vi "sn_To_Project.vi"(11 "s/n":string) -> (3 "project":string)   [LabVIEW 2011]
panel:
  in  "SerialNumber":string="[)> 06 1PLA18CB0-B40K000-F W480666 S54065 10D2047"
  # "To908.vi\nPassword:Abcd1234*\n20221117:Start new version for build Short project name to project908"
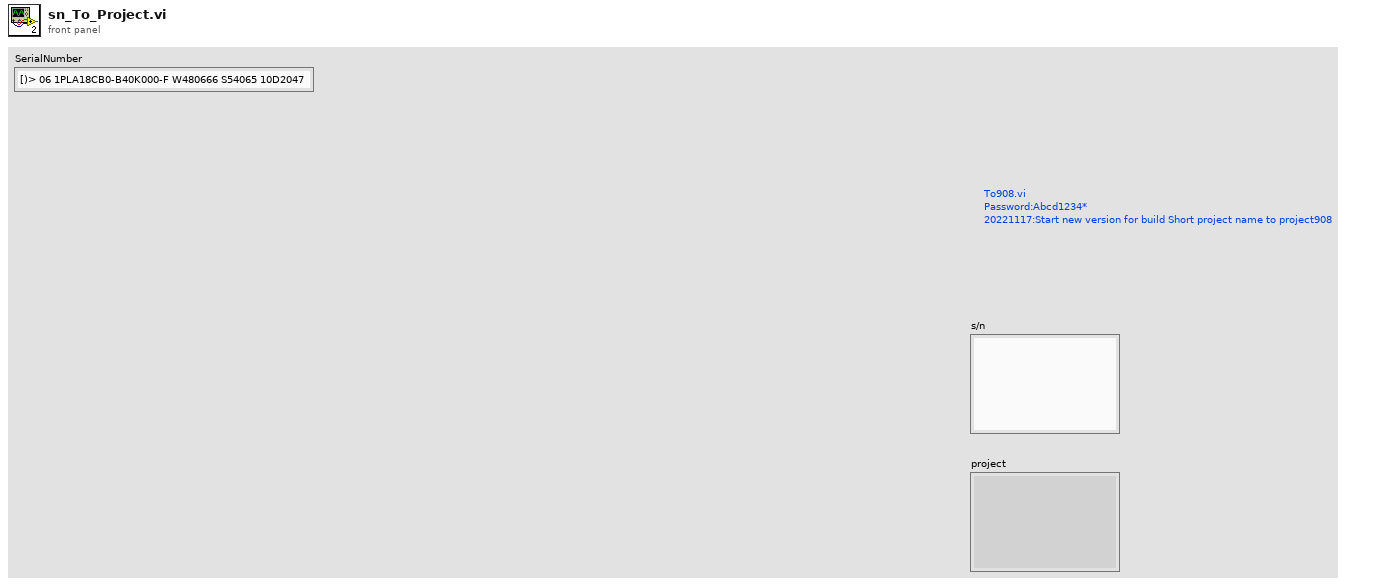
[diagram p1: front panel]
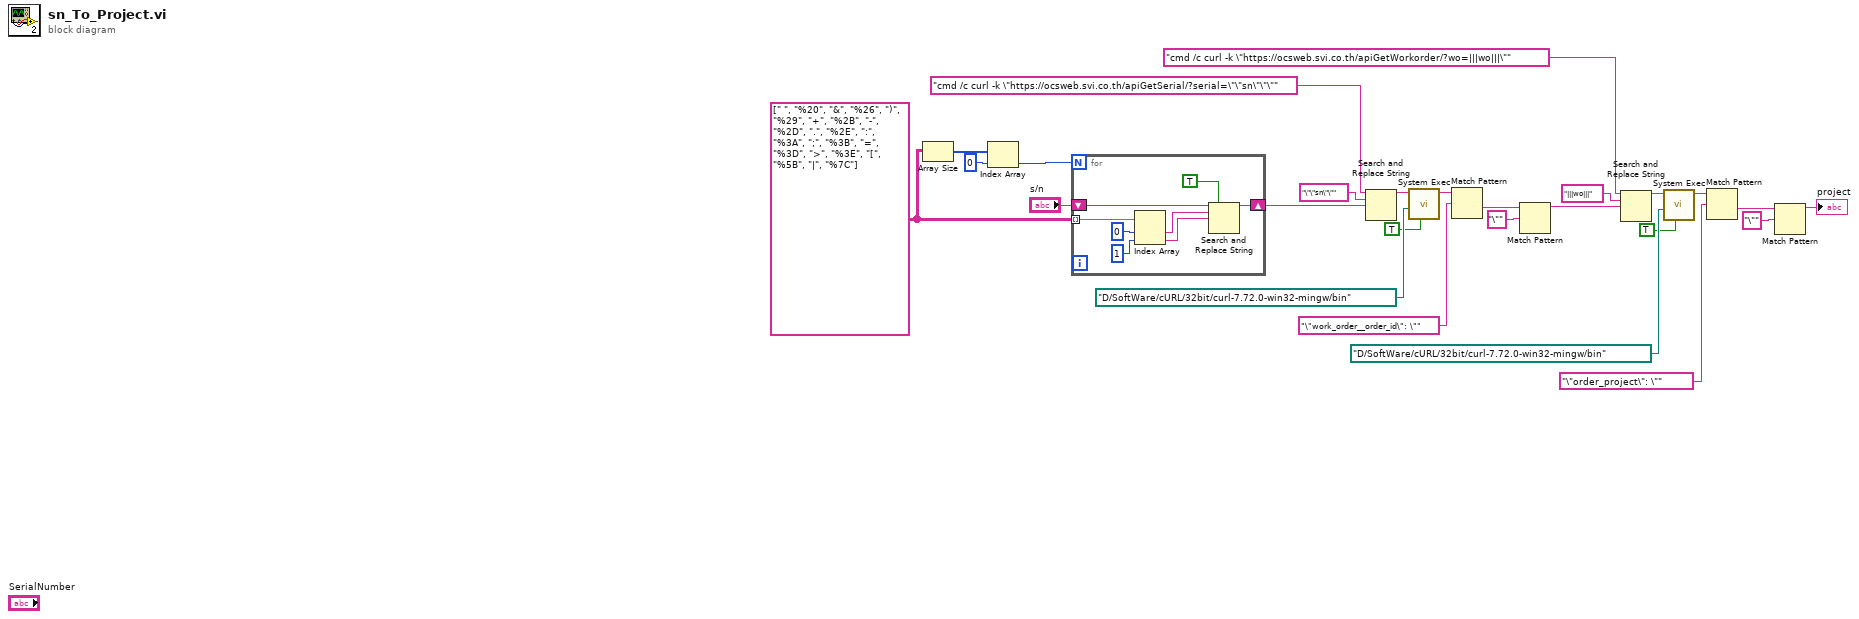
[diagram p0: block diagram]
diagram:
  w23 = string[][] [[" ", "%20"], ["&", "%26"], [")", "%29"], ["+", "%2B"], ["-", "%2D"], [".", "%2E"], [":", "%3A"], [";", "%3B"], ["=", "%3D"], [">", "%3E"], ["[", "%5B"], ["|", "%7C"]]
  n1 = Array Size(array=w23) -> (size(s)=w26:i32[])
  n2 = Index Array(array=w26, index=0) -> (element=w24:i32)
  n3 = for {
    N: w24 -> [_]
    tunnel: w23 -> [w33] mode=indexing
    shift-right: [w27] -> w20
    shift-left: "s/n" -> [w34]
    n4 = Index Array(array=w33, index #1=0 ("index"), index #2=1 ("index")) -> (element #1=w30:string, element #2=w29:string)
    n5 = Search and Replace String(replace all?=TRUE ("replace all? (F)"), input string=w34, search string=w30, replace string=w29) -> (result string=w27:string)  [unwired: 4 in, 3 out]
  }
  n6 = Search and Replace String(input string="cmd /c curl -k \"https://ocsweb.svi.co.th/apiGetSerial/?serial=\"\"sn\"\"\"" ("search string"), search string="\"\"sn\"\"", replace string=w20) -> (result string=w17:string)  [unwired: 5 in, 3 out]
  n7 = call <vilib>:"System Exec.vi"("run minimized? (F)"=TRUE, "working directory"=path "D:/SoftWare/cURL/32bit/curl-7.72.0-win32-mingw/bin", "command line"=w17) -> ("standard output"=w13:string)  [unwired: 5 in, 3 out]
  n8 = Match Pattern(string=w13, regular expression="\"work_order__order_id\": \"") -> (after substring=w15:string)  [unwired: 1 in, 3 out]
  n9 = Match Pattern(string=w15, regular expression="\"") -> (before substring=w10:string)  [unwired: 1 in, 3 out]
  n10 = Search and Replace String(input string="cmd /c curl -k \"https://ocsweb.svi.co.th/apiGetWorkorder/?wo=|||wo|||\"" ("search string"), search string="|||wo|||", replace string=w10) -> (result string=w8:string)  [unwired: 5 in, 3 out]
  n11 = call <vilib>:"System Exec.vi"("run minimized? (F)"=TRUE, "working directory"=path "D:/SoftWare/cURL/32bit/curl-7.72.0-win32-mingw/bin", "command line"=w8) -> ("standard output"=w3:string)  [unwired: 5 in, 3 out]
  n12 = Match Pattern(string=w3, regular expression="\"order_project\": \"") -> (after substring=w6:string)  [unwired: 1 in, 3 out]
  n13 = Match Pattern(string=w6, regular expression="\"") -> (before substring=→"project":string)  [unwired: 1 in, 3 out]
